vi "xmlzapis.vi"() -> ()   [LabVIEW 2021]
doc: "EasyXML Toolkit for LabVIEW version 3.0.0.170\nCopyright (c) 2016, JKI. All Rights Reserved."
panel:
  in  "XML File Path 2":path
  out "XML String":string
  in  "XML File Path":path
  in  "annotation":T1={"folder"="Funky Grooves", "filename"="Funky Grooves", "size"={"width"="", "height"="", "depth "=""}, "object"={"name"="", "pose"="", "bndbox"={"xmin"="", "ymin"="", "xmax "="", "ymax"=""}}}
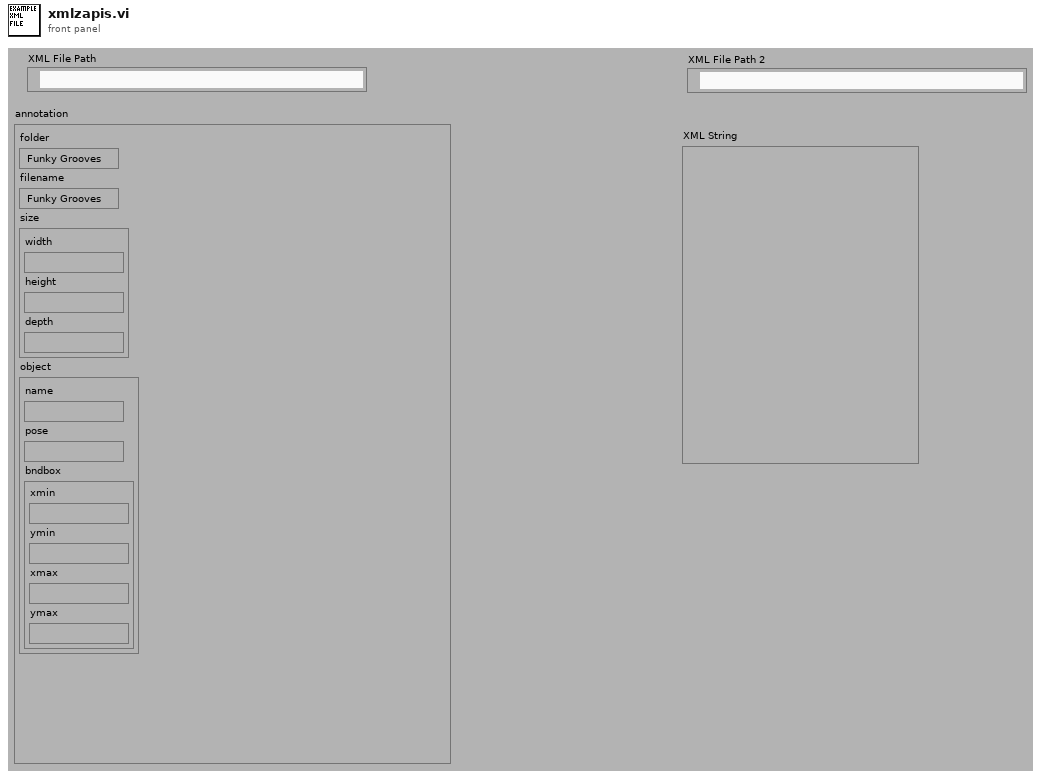
[diagram p1: front panel]
types:
  T1 = cluster{"folder":string, "filename":string, "size":cluster{"width":string, "height":string, "depth ":string}, "object":cluster{"name":string, "pose":string, "bndbox":cluster{"xmin":string, "ymin":string, "xmax ":string, "ymax":string}}}
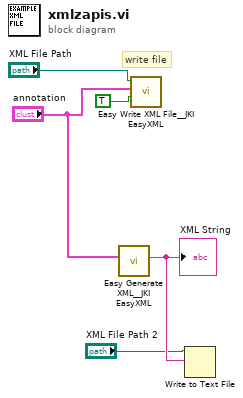
[diagram p0: block diagram]
diagram:
  # "write file"
  n1 = call <vilib>:"Easy Generate XML__JKI EasyXML.vi"("LabVIEW Data"="annotation") -> ("XML String"=w3:string)  [unwired: 9 in, 1 out]
  "XML String" <- w3
  n2 = call <vilib>:"Easy Write XML File__JKI EasyXML.vi"("Overwrite File? (false)"=TRUE, "LabVIEW Data"="annotation", "XML File Path"="XML File Path") -> ()  [unwired: 7 in, 2 out]
  n3 = Write to Text File(file (use dialog)="XML File Path 2", text=w3) -> ()  [unwired: 2 in, 3 out]
